vi "niRFUtil FWK Set Driver Validation to Database.vi"(8 "error in (no error)":errorcluster, 10 "Loaded Driver Type":T1, 11 "Driver Validation Database In":variant) -> (0 "error out":errorcluster, 3 "Driver Validation Database Out":variant)   [LabVIEW 2015, in "niRFUtil.lvlib"]
uses:
  niRFUtil.lvlib
  Includes/niRFUtil INC FWK Class Types.ctl
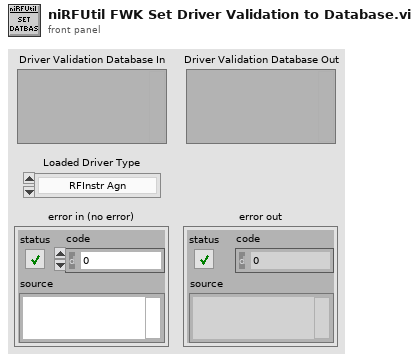
[diagram p1: front panel]
types:
  T1 = typedef "niRFUtil.lvlib/niRFUtil INC FWK Class Types.ctl" = enum16{"RFInstr Agn", "RFSAInstr", "DCPowerInstr"}
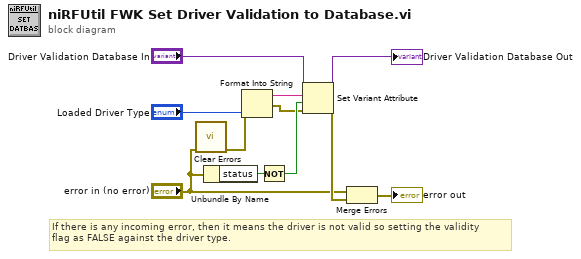
[diagram p0: block diagram]
diagram:
  # "If there is any incoming error, then it means the driver is not valid so setting the validity\nflag as FALSE against the driver type."
  n1 = call <vilib>:"Clear Errors.vi"("error in (no error)"="error in (no error)") -> ("error out"=w2:errorcluster)  [unwired: 5 in, 1 out]
  n2 = Unbundle By Name("error in (no error)") -> ("status"=w5:bool)
  n3 = Format Into String(error in=w2, "Loaded Driver Type") -> (resulting string=w7:string, error out=w1:errorcluster)  [unwired: 2 in]
  n4 = Not(x=w5) -> (.not. x?=w4:bool)
  n5 = Set Variant Attribute(Variant="Driver Validation Database In", name=w7, value=w4, error in=w1) -> (Variant out=→"Driver Validation Database Out":variant, error out=w11:errorcluster)  [unwired: 1 out]
  n6 = Merge Errors("error in (no error)", w11) -> (→"error out":errorcluster)
